vi "PushObject.vi"(8 "error in (no error)":errorcluster, 10 "Object":refnum<class "GameObject.lvclass">, 11 "PongPanel in":refnum<class "PongPanel.lvclass">) -> (0 "error out":errorcluster, 2 "Object out":refnum<class "GameObject.lvclass">, 3 "PongPanel out":refnum<class "PongPanel.lvclass">)   [LabVIEW 2019, in "RT_Game.lvlib" / "PongPanel.lvclass"]
uses:
  PongPanel.lvclass
  C:/Users/FreshBob/Dropbox/VIs/myRIO_GameConsole/RT/RT_Game/GameObject/GameObject.lvclass
  GameObject/GameObject.lvclass
  GameObject/GameObject.lvclass/GameObject.ctl
  GameObject/Read position.vi
  GameObject/Read size.vi
  GameObject/Read Velocity.vi
  RT_Game.lvlib
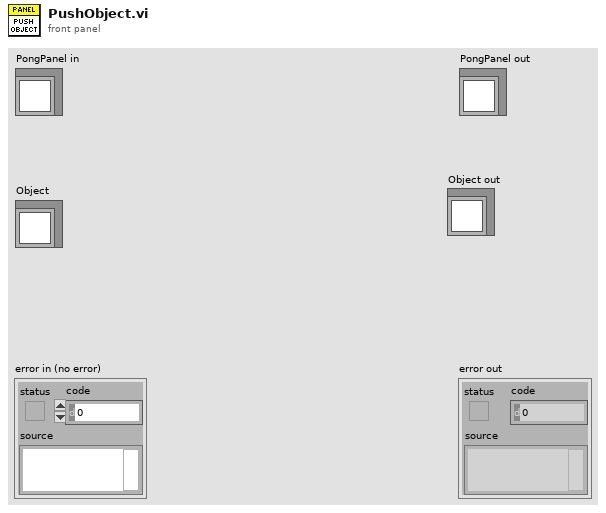
[diagram p1: front panel]
types:
  T1 = typedef "RT_Game.lvlib/Game.lvclass/Coordinate.ctl" = cluster{"x":dbl, "y":dbl}
  T2 = typedef "Velocity.ctl" = cluster{"x":dbl, "y":dbl}
  T3 = typedef "RT_Game.lvlib/Direction.ctl" = enum16{"none", "left", "right", "up", "down"}
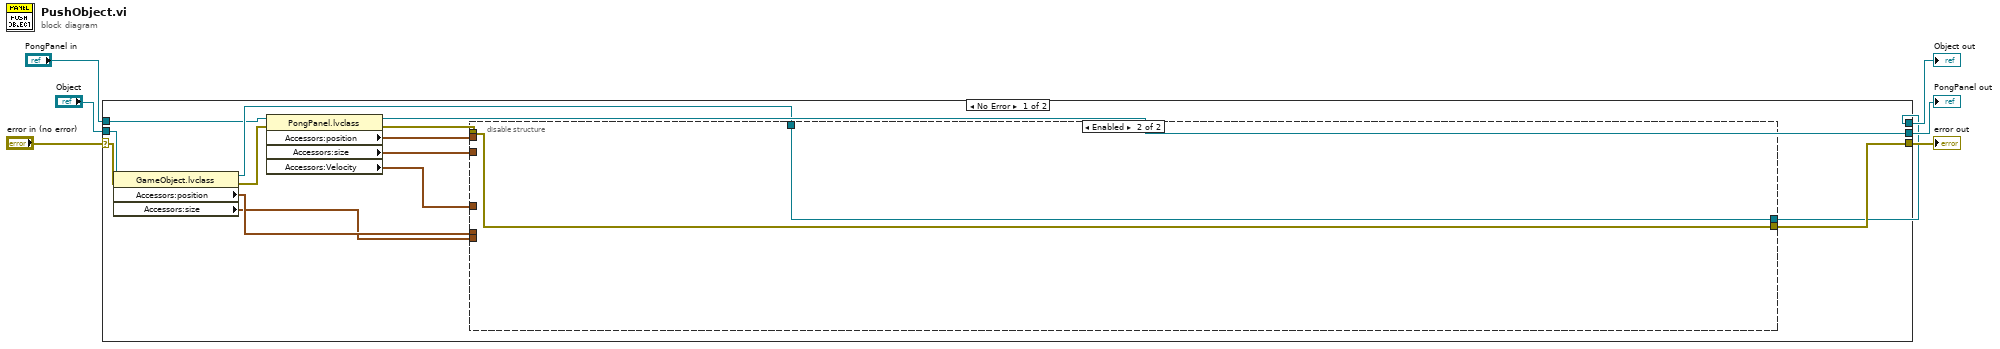
[diagram p0: block diagram]
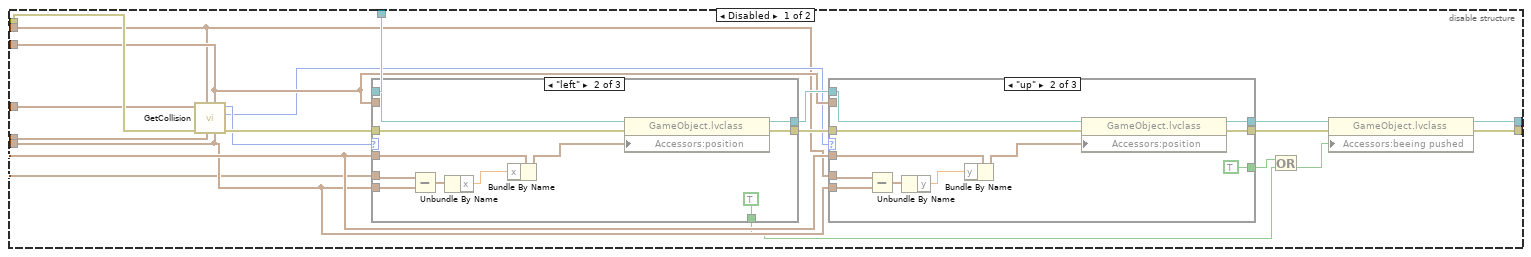
[diagram p2: hidden frame]
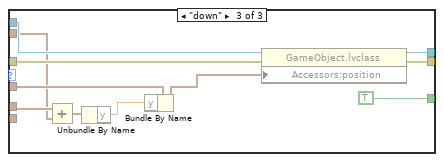
[diagram p4: hidden frame]
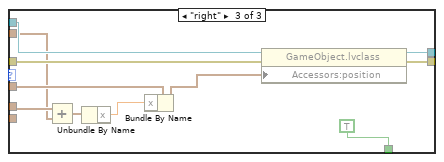
[diagram p6: hidden frame]
diagram:
  n1 = case shown="No Error" "error in (no error)" {
    selector: "error in (no error)" -> [w20 w92]
    tunnel: [w11 w92] -> w5
    tunnel: [w16 w91] -> w3
    tunnel: "PongPanel in" -> [w9 w91]
    tunnel: "Object" -> [w18 w90]
    tunnel: [w10 w90] -> w1
    frame No Error {
      n2 = property class="GameObject.lvclass"(reference=w18, error in=w20) -> (reference out=w15:refnum<class "GameObject.lvclass">, error out=w19:errorcluster, "Accessors:position"=w14:T1, "Accessors:size"=w13:T1)
      n3 = property class="PongPanel.lvclass"(reference=w9, error in=w19) -> (reference out=w16:refnum<class "PongPanel.lvclass">, error out=w17:errorcluster, "Accessors:position"=w8:T1, "Accessors:size"=w12:T1, "Accessors:Velocity"=w7:T2)
      n4 = disable-structure shown="Enabled" {
        disable-tunnel: w17 -> [w39 w89]
        disable-tunnel: w15 -> [w37 w88]
        disable-tunnel: w14 -> [w32 _]
        disable-tunnel: w13 -> [w31 _]
        disable-tunnel: w12 -> [w30 _]
        disable-tunnel: [w28 w89] -> w11
        disable-tunnel: [w26 w88] -> w10
        disable-tunnel: w8 -> [w22 _]
        disable-tunnel: w7 -> [w21 _]
        frame Disabled {
          n5 = call "GetCollision.vi"("TheirSize"=w31, "MySize"=w30, "TheirPosition"=w32, "MyPosition"=w22, "error in (no error)"=w39, "Velocity"=w21) -> ("error out"=w38:errorcluster, "direction_y"=w29:T3, "direction_x"=w36:T3)  [unwired: 3 in]
          n6 = case shown="\"left\"" w36 {
            tunnel: w38 -> [w64 w76 w87]
            tunnel: [w64 w75 w86] -> w35
            tunnel: w37 -> [w65 w74 w85]
            tunnel: [w65 w73 w84] -> w34
            tunnel: w32 -> [_ w72 w83]
            tunnel: w22 -> [_ w70 w81]
            tunnel: w31 -> [_ w69 _]
            tunnel: w30 -> [_ _ w78]
            tunnel: [_ TRUE ("x") TRUE ("x")] -> w23
            frame "none", Default {
            }
            frame "left" {
              n7 = Subtract(x=w70, y=w69) -> (x-y=w68:T1)
              n8 = Unbundle By Name(w68) -> ("x"=w67:dbl)
              n9 = Bundle By Name(cluster=w72, "x"=w67) -> (w71:T1)
              n10 = property class="GameObject.lvclass"(reference=w74, error in=w76, "Accessors:position"=w71) -> (reference out=w73:refnum<class "GameObject.lvclass">, error out=w75:errorcluster)
            }
            frame "right" {
              n11 = Add(x=w81, y=w78) -> (x+y=w80:T1)
              n12 = Unbundle By Name(w80) -> ("x"=w79:dbl)
              n13 = Bundle By Name(cluster=w83, "x"=w79) -> (w82:T1)
              n14 = property class="GameObject.lvclass"(reference=w85, error in=w87, "Accessors:position"=w82) -> (reference out=w84:refnum<class "GameObject.lvclass">, error out=w86:errorcluster)
            }
          }
          n15 = case shown="\"up\"" w29 {
            tunnel: w35 -> [w40 w52 w63]
            tunnel: [w40 w51 w62] -> w33
            tunnel: w34 -> [w41 w50 w61]
            tunnel: [w41 w49 w60] -> w27
            tunnel: w32 -> [_ w48 w59]
            tunnel: w22 -> [_ w46 w57]
            tunnel: w31 -> [_ w45 _]
            tunnel: w30 -> [_ _ w54]
            tunnel: [_ TRUE ("beeing pushed") TRUE ("beeing pushed")] -> w25
            frame "none", Default {
            }
            frame "up" {
              n16 = Subtract(x=w46, y=w45) -> (x-y=w44:T1)
              n17 = Unbundle By Name(w44) -> ("y"=w43:dbl)
              n18 = Bundle By Name(cluster=w48, "y"=w43) -> (w47:T1)
              n19 = property class="GameObject.lvclass"(reference=w50, error in=w52, "Accessors:position"=w47) -> (reference out=w49:refnum<class "GameObject.lvclass">, error out=w51:errorcluster)
            }
            frame "down" {
              n20 = Add(x=w57, y=w54) -> (x+y=w56:T1)
              n21 = Unbundle By Name(w56) -> ("y"=w55:dbl)
              n22 = Bundle By Name(cluster=w59, "y"=w55) -> (w58:T1)
              n23 = property class="GameObject.lvclass"(reference=w61, error in=w63, "Accessors:position"=w58) -> (reference out=w60:refnum<class "GameObject.lvclass">, error out=w62:errorcluster)
            }
          }
          n24 = Or(x=w25, y=w23) -> (x .or. y?=w24:bool)
          n25 = property class="GameObject.lvclass"(reference=w27, error in=w33, "Accessors:beeing pushed"=w24) -> (reference out=w26:refnum<class "GameObject.lvclass">, error out=w28:errorcluster)
        }
        frame Enabled {
        }
      }
    }
    frame Error {
    }
  }
  "error out" <- w5
  "PongPanel out" <- w3
  "Object out" <- w1
